vi "FloatConverter.vi"(11 "Reference (V)":dbl) -> (3 "String":string)   [LabVIEW 2016]
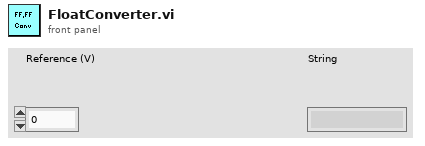
[diagram p1: front panel]
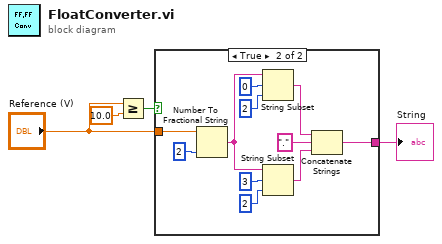
[diagram p0: block diagram]
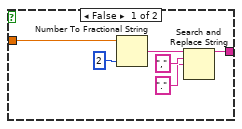
[diagram p2: hidden frame]
diagram:
  n1 = Greater Or Equal?(x="Reference (V)", y=10.0) -> (x >= y?=w2:bool)
  n2 = case shown="True" w2 {
    tunnel: "Reference (V)" -> [w9 w21]
    tunnel: [w8 w11] -> w4
    frame False {
      n3 = Number To Fractional String(number=w9, precision (6)=i16 2) -> (F-format string=w5:string)  [unwired: 2 in]
      n4 = Search and Replace String(input string=w5, search string=",", replace string="." ("search string")) -> (result string=w8:string)  [unwired: 5 in, 3 out]
    }
    frame True {
      n5 = Number To Fractional String(number=w21, precision (6)=i16 2) -> (F-format string=w12:string)  [unwired: 2 in]
      n6 = String Subset(string=w12, offset (0)=i16 0 ("precision (6)"), length (rest)=i16 2 ("precision (6)")) -> (substring=w15:string)
      n7 = String Subset(string=w12, offset (0)=i16 3 ("precision (6)"), length (rest)=i16 2 ("precision (6)")) -> (substring=w14:string)
      n8 = Concatenate Strings(w15, "." ("string"), w14) -> (w11:string)
    }
  }
  "String" <- w4
